vi "DSF.Engine.Framework.Tx.Inline.Start.vi"(8 "error in (no error)":errorcluster, 11 "Framework in":refnum<class "DSF.Engine.Framework.lvclass">) -> (0 "error out":errorcluster, 3 "Framework out":refnum<class "DSF.Engine.Framework.lvclass">)   [LabVIEW 2017, in "DSF.Engine.lvlib" / "DSF.Engine.Framework.lvclass"]
uses:
  DSF.Engine.Framework.lvclass
  DSF.Engine.Framework.lvclass/DSF.Engine.Framework.ctl
  Plugin/DSF.Engine.Plugin.lvclass/DSF.Engine.Plugin.ctl
  Timing/DSF.Engine.Timing.lvclass/DSF.Engine.Timing.ctl
  Plugin/DSF.Engine.Plugin.Get Timing.vi
  Timing/DSF.Engine.Timing.Is Active Cycle.vi
  Timing/DSF.Engine.Timing.Get Decimation.vi
  Timing/DSF.Engine.Timing.Get Offset.vi
  State/Framework State.lvclass
  Plugin/DSF.Engine.Plugin.lvclass
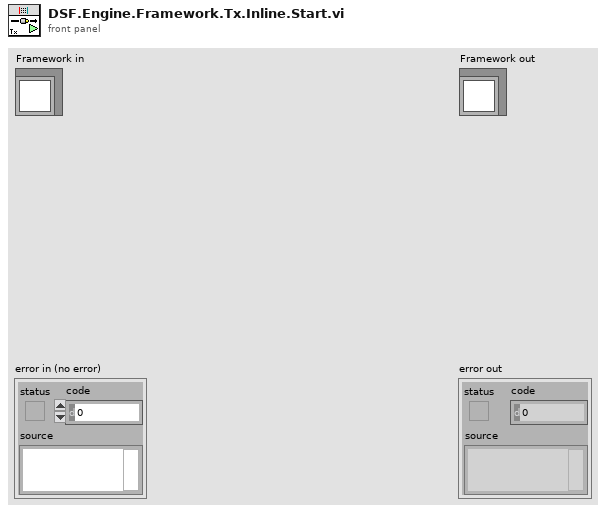
[diagram p1: front panel]
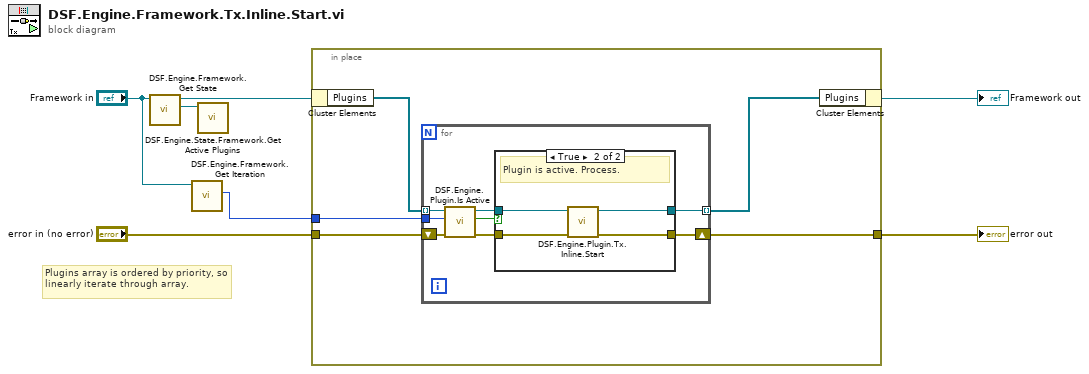
[diagram p0: block diagram]
diagram:
  # "Plugins array is ordered by priority, so linearly iterate through array."
  n1 = call "DSF.Engine.Framework.Get State.vi"("Framework in"="Framework in") -> ("State"=w5:refnum<class "Framework State.lvclass">, "Framework out"=w4:refnum<class "DSF.Engine.Framework.lvclass">)  [unwired: 9 in]
  n2 = call "DSF.Engine.Framework.Get Iteration.vi"("Framework in"="Framework in") -> ("iteration"=w1:u64)  [unwired: 9 in, 1 out]
  n3 = call "DSF.Engine.State.Framework.Get Active Plugins.vi"("Framework State in"=w5) -> ()  [unwired: 9 in, 2 out]
  n4 = in-place {
    in-place-border: "error in (no error)" -> [w12]
    in-place-border: [w11] -> w6
    in-place-border: w1 -> [w8]
    n5 = in-place-cluster #1(w4) -> ("Plugins"=w10:refnum<class "DSF.Engine.Plugin.lvclass">[])
    n6 = for {
      tunnel: w10 -> [w16] mode=indexing
      tunnel: [w19] -> w9 mode=indexing
      shift-right: [w18] -> w11
      shift-left: w12 -> [w17]
      tunnel: w8 -> [w13]
      n7 = call "DSF.Engine.Plugin.Is Active.vi"("cycle count"=w13, "Plugin in"=w16) -> ("active this cycle?"=w14:bool, "Plugin out"=w15:refnum<class "DSF.Engine.Plugin.lvclass">)  [unwired: 8 in]
      n8 = case shown="True" w14 {
        tunnel: w15 -> [w21 w25]
        tunnel: [w21 w24] -> w19
        tunnel: [w20 w22] -> w18
        tunnel: w17 -> [w20 w23]
        frame False {
          # "Plugin is not active. Skip."
        }
        frame True {
          # "Plugin is active. Process."
          n9 = call "DSF.Engine.Plugin.Tx.Inline.Start.vi"("error in (no error)"=w23, "Plugin in"=w25) -> ("error out"=w22:errorcluster, "Plugin out"=w24:refnum<class "DSF.Engine.Plugin.lvclass">)  [unwired: 8 in]
        }
      }
    }
    n10 = in-place-cluster #1("Plugins"=w9) -> (→"Framework out":refnum<class "DSF.Engine.Framework.lvclass">)
  }
  "error out" <- w6
